vi "UTILITY Plot XY Build Data.vi"(7 "Reset":bool, 9 "Data Array":dbl[](array[numeric]), 10 "Time (s)":dbl, 11 "Max Array Size":i32) -> (2 "Plot Data":cluster{dbl[], dbl[]}[](array[cluster]))   [LabVIEW 2016]
panel:
  out "Array":dbl[][](array[numeric])
  out "transposed array":dbl[][](array[numeric])
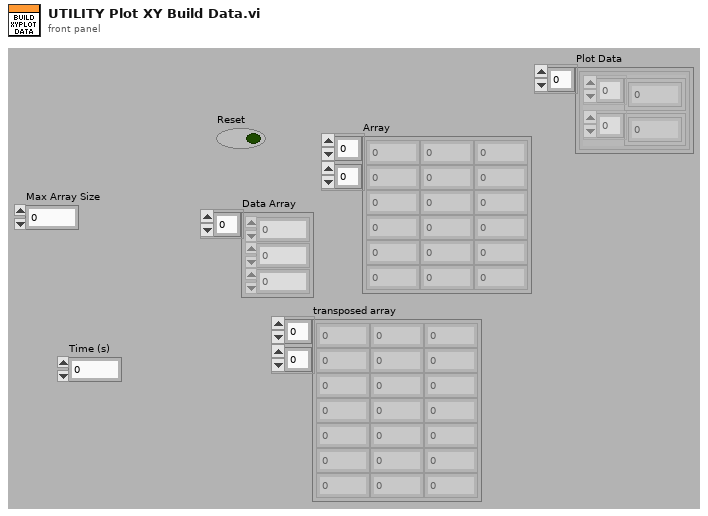
[diagram p1: front panel]
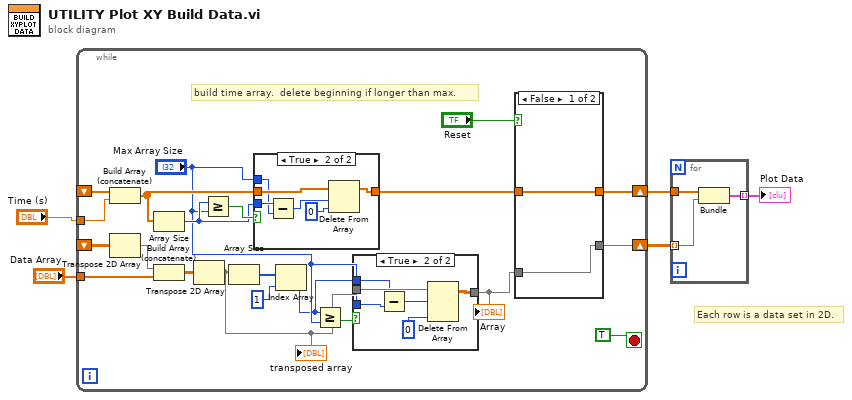
[diagram p0: block diagram]
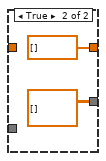
[diagram p3: hidden frame]
diagram:
  # "Each row is a data set in 2D."
  n1 = while {
    shift-right: [w21] -> w3
    shift-left: _ -> [w22]
    tunnel: "Time (s)" -> [w18]
    tunnel: "Data Array" -> [w17]
    shift-right: [w16] -> w2
    shift-left: _ -> [w14]
    stop <- TRUE stop-if-true
    # "build time array.  delete beginning if longer than max."
    n2 = Build Array (concatenate)(w22, w18) -> (w24:dbl[])
    n3 = Transpose 2D Array(2D array=w14) -> (transposed array=w13:dbl[][])
    n4 = Array Size(array=w24) -> (size(s)=w23:i32)
    n5 = Build Array (concatenate)(w13, w17) -> (w15:dbl[][])
    n6 = Transpose 2D Array(2D array=w15) -> (transposed array=w10:dbl[][])
    "transposed array" <- w10
    n7 = Greater Or Equal?(x=w23, y="Max Array Size") -> (x >= y?=w25:bool)
    n8 = Array Size(array=w10) -> (size(s)=w12:i32[])
    n9 = case shown="True" w25 {
      tunnel: [w38 w44] -> w20
      tunnel: w24 -> [w38 w43]
      tunnel: w23 -> [_ w40]
      tunnel: "Max Array Size" -> [_ w39]
      frame False {
      }
      frame True {
        n10 = Subtract(x=w40, y=w39) -> (x-y=w41:i32)
        n11 = Delete From Array(array=w43, length=w41, index=0) -> (array with subset deleted=w44:dbl[])  [unwired: 1 out]
      }
    }
    n12 = Index Array(array=w12, index=1) -> (element=w6:i32)
    n13 = Greater Or Equal?(x=w6, y="Max Array Size") -> (x >= y?=w9:bool)
    n14 = case shown="True" w9 {
      tunnel: [w27 w33] -> w8
      tunnel: w10 -> [w27 w32]
      tunnel: "Max Array Size" -> [_ w30]
      tunnel: w6 -> [_ w29]
      frame False {
      }
      frame True {
        n15 = Subtract(x=w29, y=w30) -> (x-y=w31:i32)
        n16 = Delete From Array(array=w32, length=w31, index (col)=0 ("index")) -> (array with subset deleted=w33:dbl[][])  [unwired: 1 in, 1 out]
      }
    }
    "Array" <- w8
    n17 = case shown="False" "Reset" {
      tunnel: [w35 dbl[] []] -> w21
      tunnel: w20 -> [w35 _]
      tunnel: [w34 dbl[][] []] -> w16
      tunnel: w8 -> [w34 _]
      frame False {
      }
      frame True {
      }
    }
  }
  n18 = for {
    tunnel: w3 -> [w47]
    tunnel: [w46] -> w1 mode=indexing
    tunnel: w2 -> [w45] mode=indexing
    n19 = Bundle(w47, w45) -> (w46:cluster{dbl[], dbl[]})  [unwired: 1 out]
  }
  "Plot Data" <- w1
